vi "Generate 2D scan Waveform.vi"(8 "error in (no error)":errorcluster, 11 "System Parameters [In]":T1={"Optical Parameters"={"Obj. Focal Length [mm]"=0.0, "Scan Lens EFL[mm]"=0.0, "Tube Lens EFL[mm]"=0.0, "Galvo V Range (+/-)"=0.0, "Galvo Max Half Angle [Deg]"=0.0, "Max Galvo Range[%]"=0.0}, "Vibratome"={"Z Bottom [mm]"=0.0, "Pre Cut Dwell [s]"=0.0, "Blade Frequency [RPM]"=0, "Slice Speed [mm/s]"=0.0, "Post Cut Dwell [s]"=0.0, "Ramp Time [s]"=0.0, "Start X [mm]"=0.0, "Start Y [mm]"=0.0, "Slice Length [mm]"=0.0, "Slice Axis"=enum."Y Axis", "Controller VISA Ref"="COM4"}, "Table Stages"={"X Stage"={"Position"=0.0, "Is.Enabled?"=FALSE, "Is.Connected?"=FALSE, "Device SN"="45876539", "AccelerationMaximum"=0.0, "VelocityMaximum"=0.0, "Acceleration"=0.0, "Velocity"=0.0, "waitTimeout (ms)"=0, "Model"=enum."None", "Is.Homed?"=FALSE}, "Y Stage"={"Position"=0.0, "Is.Enabled?"=FALSE, "Is.Connected?"=FALSE, "Device SN"="45876539", "AccelerationMaximum"=0.0, "VelocityMaximum"=0.0, "Acceleration"=0.0, "Velocity"=0.0, "waitTimeout (ms)"=0, "Model"=enum."None", "Is.Homed?"=FALSE}, "Z Stage"={"Position"=0.0, "Is.Enabled?"=FALSE, "Is.Connected?"=FALSE, "Device SN"="45876539", "AccelerationMaximum"=0.0, "VelocityMaximum"=0.0, "Acceleration"=0.0, "Velocity"=0.0, "waitTimeout (ms)"=0, "Model"=enum."None", "Is.Homed?"=FALSE}}, "Imaging Parameter"={"Raster Scan Direction"=enum."Uni Directional", "Pixel Dwell Time [Clock Cycles]"=0, "Flyback Time [Clock Cycles]"=0, "XY Center [um]"={"X"=1.0, "Y"=1.0}, "Pixel Step Size [um]"=1.0, "XY Image Size"=enum."256 x 256", "Custom"=FALSE, "Custom Size"={"X"=1, "Y"=1}, "Line Averages"=1}} {"Imaging Parameter"."Line Averages" min=1 max=30 step=1; "Imaging Parameter"."Flyback Time [Clock Cycles]" max=10 step=1; "Imaging Parameter"."Pixel Step Size [um]" min=0.0 max=10.0 step=0.01; "Imaging Parameter"."Custom Size"."Y" min=1 max=30 step=1; "Imaging Parameter"."Custom Size"."X" min=1 max=30 step=1; "Imaging Parameter"."XY Center [um]"."Y" min=1.0 max=30.0 step=1.0; "Imaging Parameter"."XY Center [um]"."X" min=1.0 max=30.0 step=1.0; "Imaging Parameter"."Pixel Dwell Time [Clock Cycles]" max=10 step=1}) -> (0 "error out":errorcluster, 1 "Y":dbl[](graph), 2 "Digital Line Acq":bool[](array[boolean]), 3 "XY":dbl[][](array[numeric]), 5 "X":dbl[](graph), 7 "DO":i16[](graph))   [LabVIEW 2018]
uses:
  Controls/System Parameters.ctl
  Controls/Optical Parameters.ctl
  Controls/Vibratome Parameters.ctl
  Controls/Translation Stage Parameters.ctl
  Hardware Mfg/Thorlabs Translation Stages/Controls/Translation Stage Cluster.ctl
  Controls/Translation Stage Types.ctl
  Controls/Imaging Parameters.ctl
  Controls/Scan Direction.ctl
panel:
  out "dt":dbl
  # "X"
  # "X"
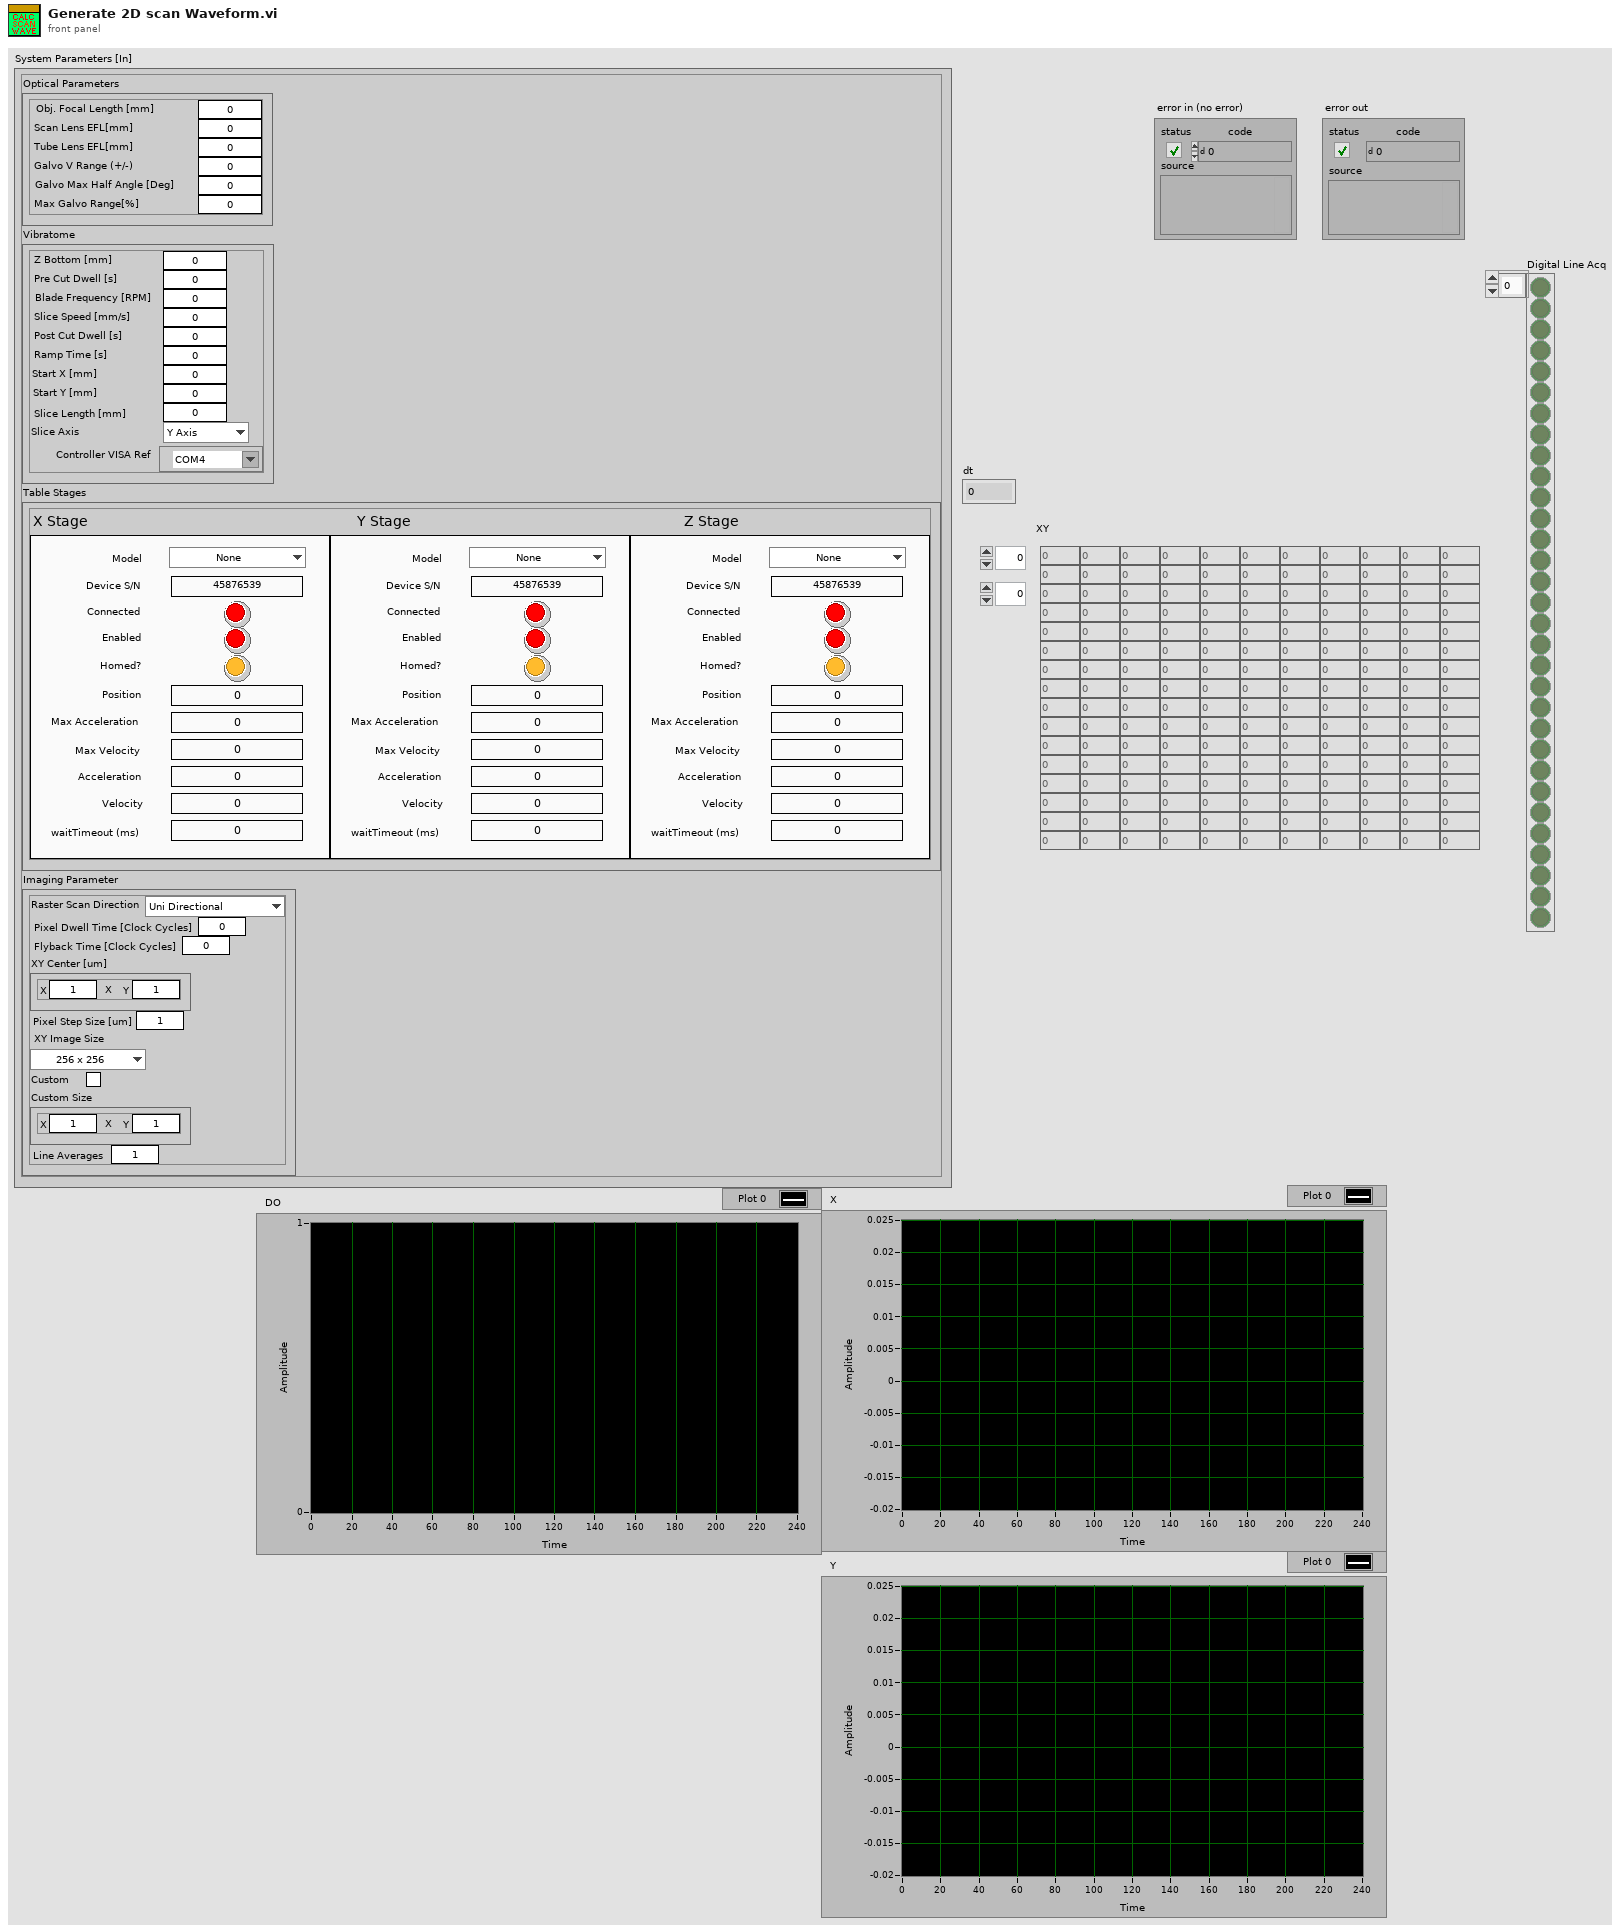
[diagram p1: front panel]
types:
  T1 = typedef "System Parameters.ctl" = cluster{"Optical Parameters":T2, "Vibratome":T3, "Table Stages":T4, "Imaging Parameter":T7}
  T2 = typedef "Optical Parameters.ctl" = cluster{"Obj. Focal Length [mm]":dbl, "Scan Lens EFL[mm]":dbl, "Tube Lens EFL[mm]":dbl, "Galvo V Range (+/-)":dbl, "Galvo Max Half Angle [Deg]":dbl, "Max Galvo Range[%]":dbl}
  T3 = typedef "Vibratome Parameters.ctl" = cluster{"Z Bottom [mm]":dbl, "Pre Cut Dwell [s]":dbl, "Blade Frequency [RPM]":u16, "Slice Speed [mm/s]":dbl, "Post Cut Dwell [s]":dbl, "Ramp Time [s]":dbl, "Start X [mm]":dbl, "Start Y [mm]":dbl, "Slice Length [mm]":dbl, "Slice Axis":enum16{"X Axis", "Y Axis", "Z Axis"}, "Controller VISA Ref":refnum<visa-resource-name>}
  T4 = typedef "Translation Stage Parameters.ctl" = cluster{"X Stage":T5, "Y Stage":T5, "Z Stage":T5}
  T5 = typedef "Translation Stage Cluster.ctl" = cluster{"Position":dbl, "Is.Enabled?":bool, "Is.Connected?":bool, "Device SN":string, "AccelerationMaximum":dbl, "VelocityMaximum":dbl, "Acceleration":dbl, "Velocity":dbl, "waitTimeout (ms)":i32, "Model":T6, "Is.Homed?":bool}
  T6 = typedef "Translation Stage Types.ctl" = enum16{"None", "Thorlabs LTS", "Thorlabs MLJ"}
  T7 = typedef "Imaging Parameters.ctl" = cluster{"Raster Scan Direction":T8, "Pixel Dwell Time [Clock Cycles]":u16, "Flyback Time [Clock Cycles]":u16, "XY Center [um]":cluster{"X":dbl, "Y":dbl}, "Pixel Step Size [um]":dbl, "XY Image Size":enum16{"32 x 32", "64 x 64", "128 x 128", "256 x 256", "512 x 512", "1024 x 1024", "2048 x 2048"}, "Custom":bool, "Custom Size":cluster{"X":u16, "Y":u16}, "Line Averages":u8}
  T8 = typedef "Scan Direction.ctl" = enum16{"Uni Directional", "Bi Directional", "None"}
  T9 = enum16{"32 x 32", "64 x 64", "128 x 128", "256 x 256", "512 x 512", "1024 x 1024", "2048 x 2048"}
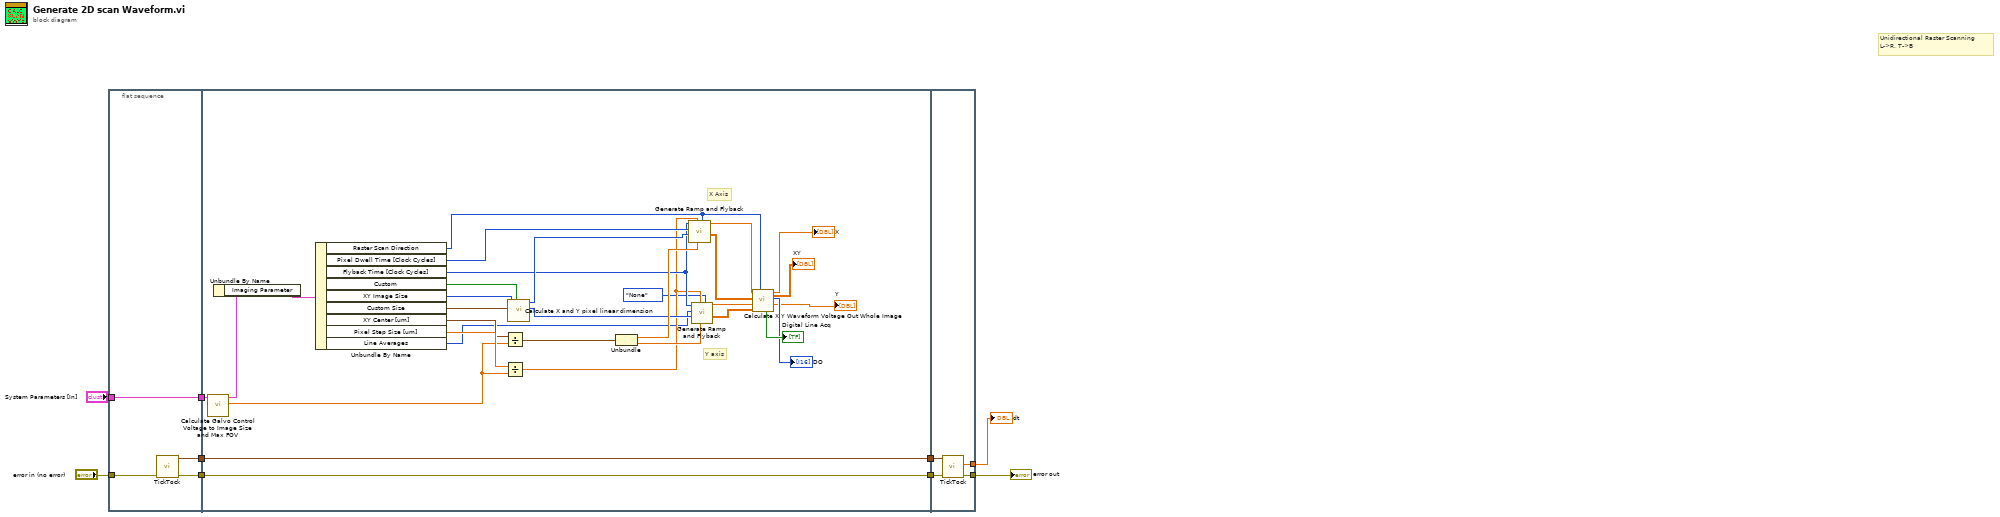
[diagram p0: block diagram]
diagram:
  # "Unidirectional Raster Scanning\nL->R, T->B"
  n1 = flat-sequence {
    tunnel: "System Parameters [In]" -> [w13]
    tunnel: [w13] -> w8
    tunnel: [w12] -> w6
    tunnel: [w11] -> w4
    tunnel: "error in (no error)" -> [w10]
    tunnel: w8 -> [w43]
    tunnel: [w20] -> w7
    tunnel: w6 -> [w20]
    tunnel: [w19] -> w5
    tunnel: w4 -> [w19]
    tunnel: w7 -> [w48]
    tunnel: w5 -> [w47]
    tunnel: [w46] -> w3
    tunnel: [w45] -> w1
    frame #0 {
      n2 = call "TickTock.vi"("Error In"=w10) -> ("Error Out"=w12:errorcluster, "Current Time (Out)"=w11:timestamp)  [unwired: 8 in, 1 out]
    }
    frame #1 {
      # "X Axis"
      # "Y axis"
      n3 = call "Calculate Galvo Control Voltage to Image Size and Max FOV.vi"("System Parameters [In]"=w43) -> ("Galvo [um/V]"=w35:dbl, "System Parameters [Out]"=w42:T1)  [unwired: 7 in, 2 out]
      n4 = Unbundle By Name(w42) -> ("Imaging Parameter"=w44:T7)
      n5 = Unbundle By Name(w44) -> ("Raster Scan Direction"=w21:T8, "Pixel Dwell Time [Clock Cycles]"=w33:u16, "Flyback Time [Clock Cycles]"=w31:u16, "Custom"=w38:bool, "XY Image Size"=w41:T9, "Custom Size"=w40:cluster{"X":u16, "Y":u16}, "XY Center [um]"=w36:cluster{"X":dbl, "Y":dbl}, "Pixel Step Size [um]"=w37:dbl, "Line Averages"=w27:u8)
      n6 = Divide(x=w36, y=w35) -> (x/y=w39:cluster{"X":dbl, "Y":dbl})
      n7 = Divide(x=w37, y=w35) -> (x/y=w28:dbl)
      n8 = call "Calculate X and Y pixel linear dimension.vi"("Imaging Parameter.Custom"=w38, "Custom Size"=w40, "XY Image Resolution"=w41) -> ("Y Px Dim (HFOV)"=w30:u16, "X Px Dim (HFOV)"=w32:u16)  [unwired: 5 in, 2 out]
      n9 = Unbundle(w39) -> ("X"=w34:dbl, "Y"=w29:dbl)
      n10 = call "Generate Ramp and Flyback.vi"("Raster Scan Direction"=w21, "FOV Center (V)"=w34, "Galvo Step Size Voltages (px/V)"=w28, "Px Dim (HFOV)"=w32, "Pixel Dwell Time [Clock Cycles]"=w33, "Flyback Time [Clock Cycles]"=w31) -> ("Flyback"=w24:dbl[][], "Waveform Graph"=w22:dbl[])  [unwired: 3 in, 1 out]
      n11 = call "Generate Ramp and Flyback.vi"("Raster Scan Direction"=Scan_Direction."None", "FOV Center (V)"=w29, "Galvo Step Size Voltages (px/V)"=w28, "Px Dim (HFOV)"=w30, "Pixel Dwell Time [Clock Cycles]"=w27, "Flyback Time [Clock Cycles]"=w31) -> ("Flyback"=w25:dbl[][], "Waveform Graph"=w23:dbl[])  [unwired: 3 in, 1 out]
      n12 = call "Calculate X Y Waveform Voltage Out Whole Image.vi"("Raster Scan Direction"=w21, "Y Flyback"=w25, "Y Waveform"=w23, "X Flyback"=w24, "X Waveform"=w22) -> ("Y Waveform Out"=→"Y":dbl[], "DO"=→"DO":i16[], "X Waveform Out"=→"X":dbl[], "Digital Line Acq"=→"Digital Line Acq":bool[], "XY Waveform Out"=→"XY":dbl[][])  [unwired: 2 in]
    }
    frame #2 {
      n13 = call "TickTock.vi"("Error In"=w48, "Current Time (In)"=w47) -> ("Error Out"=w45:errorcluster, "dt"=w46:dbl)  [unwired: 7 in, 1 out]
    }
  }
  "dt" <- w3
  "error out" <- w1
